vi "ZplInt2String.vi"(1 "字符":string="0", 2 "Int":i32) -> (0 "outString":string)   [LabVIEW 2018]
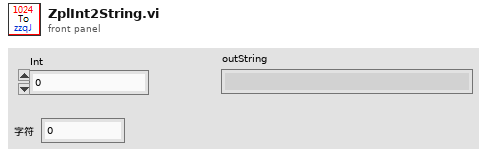
[diagram p1: front panel]
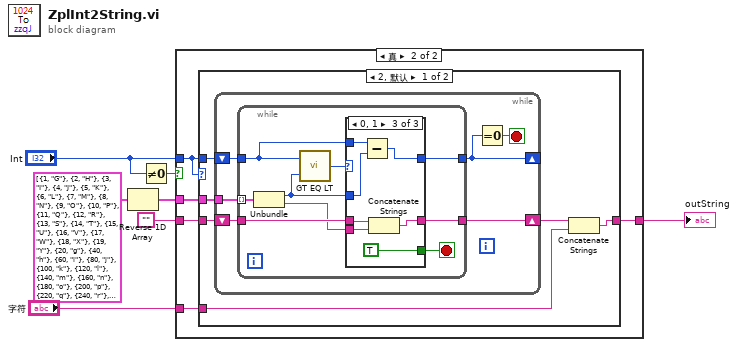
[diagram p0: block diagram]
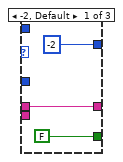
[diagram p3: hidden frame]
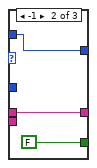
[diagram p4: hidden frame]
diagram:
  n1 = Reverse 1D Array(array=cluster{i32, string}[] [{1, "G"}, {2, "H"}, {3, "I"}, {4, "J"}, {5, "K"}, {6, "L"}, {7, "M"}, {8, "N"}, {9, "O"}, {10, "P"}, {11, "Q"}, {12, "R"}, {13, "S"}, {14, "T"}, {15, "U"}, {16, "V"}, {17, "W"}, {18, "X"}, {19, "Y"}, {20, "g"}, {40, "h"}, {60, "i"}, {80, "j"}, {100, "k"}, {120, "l"}, {140, "m"}, {160, "n"}, {180, "o"}, {200, "p"}, {220, "q"}, {240, "r"}, {260, "s"}, {280, "t"}, {300, "u"}, {320, "v"}, {340, "w"}, {360, "x"}, {380, "y"}, {400, "z"}]) -> (reversed array=w6:cluster{i32, string}[])
  n2 = Not Equal To 0?(x="Int") -> (x != 0?=w2:bool)
  n3 = case shown="真" w2 {
    tunnel: w6 -> [_ w13]
    tunnel: "" -> [w8 w12]
    tunnel: [w8 w11] -> w4
    tunnel: "Int" -> [_ w10]
    tunnel: "字符" -> [_ w9]
    frame False {
    }
    frame True {
      n4 = case shown="2, 默认" w10 {
        tunnel: w13 -> [w19 _]
        tunnel: w10 -> [w18 _]
        tunnel: w12 -> [w17 _]
        tunnel: [w15 w48] -> w11
        tunnel: w9 -> [w14 w48]
        frame 2, Default {
          n5 = while {
            tunnel: w19 -> [w25]
            shift-right: [w21] -> _
            shift-left: w18 -> [w24]
            shift-right: [w22] -> w16
            shift-left: w17 -> [w23]
            stop <- w20 stop-if-true
            n6 = while {
              tunnel: w25 -> [w34] mode=indexing
              tunnel: w24 -> [w32]
              tunnel: [w28] -> w21
              tunnel: w23 -> [w30]
              tunnel: [w29] -> w22
              stop <- w26 stop-if-true
              n7 = Unbundle(w34) -> (w31:i32, w27:string)
              n8 = call "GT EQ LT.vi"("基准"=w31, "in"=w32) -> ("out"=w33:i32)
              n9 = case shown="0, 1" w33 {
                tunnel: w32 -> [_ w40 w47]
                tunnel: [-2 ("in") w40 w45] -> w28
                tunnel: w31 -> [_ _ w46]
                tunnel: w30 -> [w36 w39 w44]
                tunnel: [w36 w39 w42] -> w29
                tunnel: w27 -> [_ _ w43]
                tunnel: [FALSE FALSE TRUE] -> w26
                frame -2, Default {
                }
                frame -1 {
                }
                frame 0, 1 {
                  n10 = Subtract(x=w47, y=w46) -> (x-y=w45:i32)
                  n11 = Concatenate Strings(w44, w43) -> (w42:string)
                }
              }
            }
            n12 = Equal To 0?(x=w21) -> (x = 0?=w20:bool)
          }
          n13 = Concatenate Strings(w16, w14) -> (w15:string)
        }
        frame 1 {
        }
      }
    }
  }
  "outString" <- w4
